vi "Set Bit.vi"(0 "OWEN HMI in":refnum<class "OWEN HMI.lvclass">, 7 "bit":T1, 9 "value":bool, 11 "error in (no error)":errorcluster) -> (4 "OWEN HMI out":refnum<class "OWEN HMI.lvclass">, 15 "error out":errorcluster)   [LabVIEW 2019, in "OWEN HMI.lvclass"]
uses:
  OWEN HMI.lvclass
  Bit.ctl
  OWEN HMI.lvclass/OWEN HMI.ctl
  Words.ctl
  0786c6a3-239e-48e0-a0ea-456b97e7ad3c.vi
  <vilib>/NI/Modbus Library/API/Master/Modbus Master.lvclass
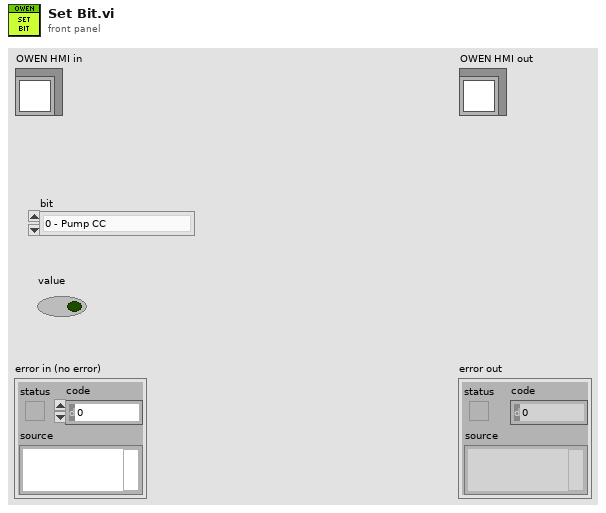
[diagram p1: front panel]
types:
  T1 = typedef "OWEN HMI.lvclass/Bit.ctl" = enum16{"0 - Pump CC", "1 - Pump SO", "2 - Alarm", "3 - Warning", "4 - DUT", "5 - CHMBR"}
  T2 = typedef "OWEN HMI.lvclass/Words.ctl" = enum16{"0 - Bits", "1 - Level CC", "2 - Temp CC", "3 - Level SO", "4 - Temp SO"}
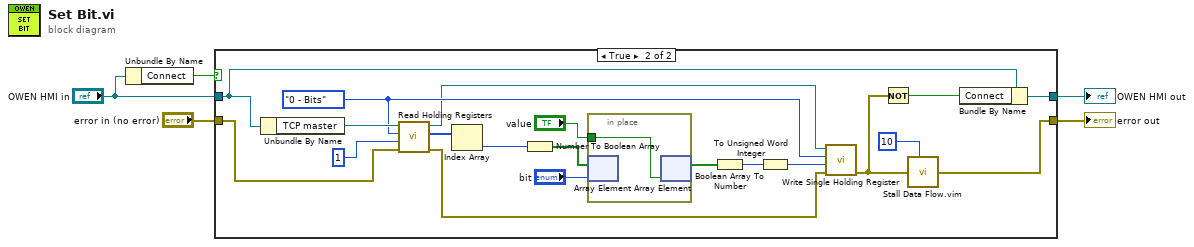
[diagram p0: block diagram]
diagram:
  n1 = Unbundle By Name("OWEN HMI in") -> ("Connect"=w1:bool)
  n2 = case shown="True" w1 {
    tunnel: "error in (no error)" -> [w6 w27]
    tunnel: [w6 w12] -> w4
    tunnel: "OWEN HMI in" -> [w7 w8]
    tunnel: [w7 w11] -> w3
    frame False {
    }
    frame True {
      w23 = Words."0 - Bits" ("Word")
      n3 = Unbundle By Name(w8) -> ("TCP master"=w26:refnum<class "Modbus Master.lvclass">)
      n4 = call-dynamic "Read Holding Registers.vi"("error in"=w27, "number of inputs"=u16 1, "starting address"=w23, "Modbus master in"=w26) -> ("error out"=w14:errorcluster, "register values"=w20:u16[], "Modbus master out"=w21:refnum<class "Modbus Master.lvclass">)  [unwired: 5 in]
      n5 = Index Array(array=w20) -> (element=w19:u16)  [unwired: 1 in]
      n6 = Number To Boolean Array(number=w19) -> (Boolean array=w18:bool[])
      n7 = in-place {
        in-place-border: "value" -> [w28]
        n8 = in-place-array #1(w18, "bit") -> ()  [unwired: 1 out]
        n9 = in-place-array #1(w28) -> (w17:bool[])  [unwired: 1 out]
      }
      n10 = Boolean Array To Number(Boolean array=w17) -> (number=w16:u32)
      n11 = To Unsigned Word Integer(number=w16) -> (unsigned 16bit integer=w15:u16)
      n12 = call-dynamic "Write Single Holding Register.vi"("error in"=w14, "register to write"=w15, "address"=w23, "Modbus master in"=w21) -> ("error out"=w10:errorcluster)  [unwired: 6 in, 1 out]
      n13 = Not(x=w10) -> (.not. x?=w9:bool)
      n14 = call "Stall Data Flow.vim"("value in"=w10, "milliseconds to wait"=u32 10) -> ("value out"=w12:errorcluster)  [unwired: 1 out]
      n15 = Bundle By Name(cluster=w8, "Connect"=w9) -> (w11:refnum<class "OWEN HMI.lvclass">)
    }
  }
  "error out" <- w4
  "OWEN HMI out" <- w3
